vi "Scale Period.vi"(0 "period (S)":fxp<+,32,16> format="%#.5g", 9 "sample rate (S/s)":dbl format="%#_6p", 11 "error in (no error)":errorcluster) -> (4 "period (s)":dbl, 8 "frequency (Hz)":dbl format="%#_6p", 15 "error out":errorcluster)   [LabVIEW 2020, in "NI_FpgaMspHost.lvlib"]
doc: "Converts the period output, expressed in samples, from the Analog Period Measurement Express VI to a period in units of seconds using the sample rate you specify. This VI also returns the frequency of the measurement in hertz using the sample rate you specify. Use the Scale Period VI in a host VI."
uses:
  <vilib>/rvi/Analysis/host/Public/NI_FpgaMspHost.lvlib
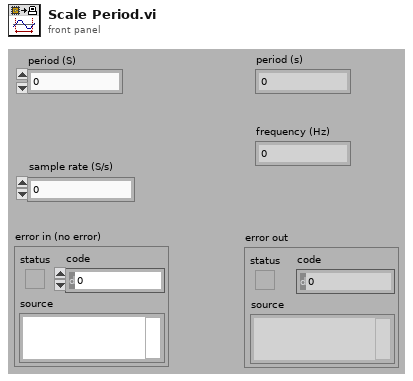
[diagram p1: front panel]
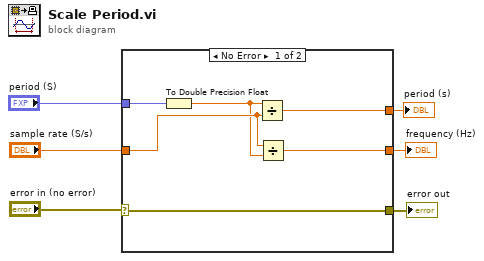
[diagram p0: block diagram]
diagram:
  n1 = case shown="No Error" "error in (no error)" {
    selector: "error in (no error)" -> [w7 w13]
    tunnel: "period (S)" -> [w12 _]
    tunnel: "sample rate (S/s)" -> [w11 _]
    tunnel: [w9 _] -> w4
    tunnel: [w8 _] -> w3
    tunnel: [w7 w13] -> w1
    frame No Error {
      n2 = To Double Precision Float(number=w12) -> (double precision float=w10:dbl)
      n3 = Divide(x=w10, y=w11) -> (x/y=w8:dbl)
      n4 = Divide(x=w11, y=w10) -> (x/y=w9:dbl)
    }
    frame Error {
    }
  }
  "period (s)" <- w3
  "frequency (Hz)" <- w4
  "error out" <- w1
